vi "DAQmx Create Channel (AI-Strain-Rosette Strain Gage).vi"(0 "task in":refnum<k21>, 1 "maximum value":dbl=0.001 format="%0.7f", 2 "minimum value":dbl=-0.001 format="%0.7f", 5 "physical channels":tag, 7 "name to assign":string, 9 "rosette configuration":T1={"rosette type"=15968, "gage orientation"=0.0, "rosette measurements"=[15971]} {"rosette measurements" items=["Principal Strain 1"=15971, "Principal Strain 2"=15972, "Principal Strain Angle"=15973, "Cartesian Strain X"=15974, "Cartesian Strain Y"=15975, "Cartesian Shear Strain XY"=15976, "Maximum Shear Strain"=15977, "Maximum Shear Strain Angle"=15978]; "rosette type" items=["Rectangular Rosette"=15968, "Delta Rosette"=15969, "Tee Rosette"=15970]}, 11 "error in":errorcluster, 13 "bridge information":T2={"strain configuration"=10271, "lead wire resistance"=0.0, "voltage excitation source"=10200, "voltage excitation value"=2.5} {"voltage excitation source" items=["Internal"=10200, "External"=10167, "None"=10230]; "voltage excitation value" format="%0.2f"; "lead wire resistance" format="%0.2f"; "strain configuration" items=["Full Bridge I"=10183, "Full Bridge II"=10184, "Full Bridge III"=10185, "Half Bridge I"=10188, "Half Bridge II"=10189, "Quarter Bridge I"=10271, "Quarter Bridge II"=10272]}, 14 "strain gage information":T3={"gage factor"=2.0, "nominal gage resistance"=350.0, "poisson ratio"=0.3} {"poisson ratio" format="%0.2f"; "nominal gage resistance" format="%0.2f"; "gage factor" format="%0.2f"}) -> (4 "task out":refnum<k21>, 15 "error out":errorcluster)   [LabVIEW 2020]
doc: "Creates channels to measure two-dimensional strain using a rosette strain gage."
uses:
  nilvaiu.dll
panel:
  # "input limits"
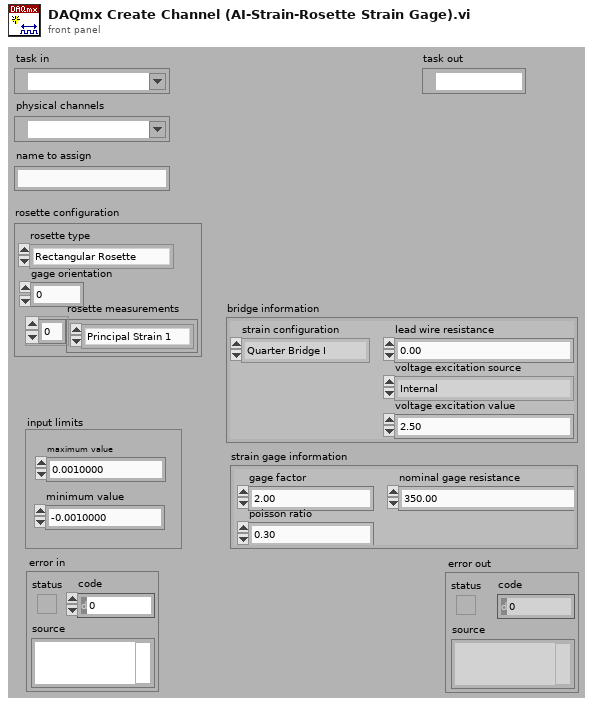
[diagram p1: front panel]
types:
  T1 = cluster{"rosette type":i32, "gage orientation":dbl, "rosette measurements":i32[]}
  T2 = cluster{"strain configuration":i32, "lead wire resistance":dbl, "voltage excitation source":i32, "voltage excitation value":dbl}
  T3 = cluster{"gage factor":dbl, "nominal gage resistance":dbl, "poisson ratio":dbl}
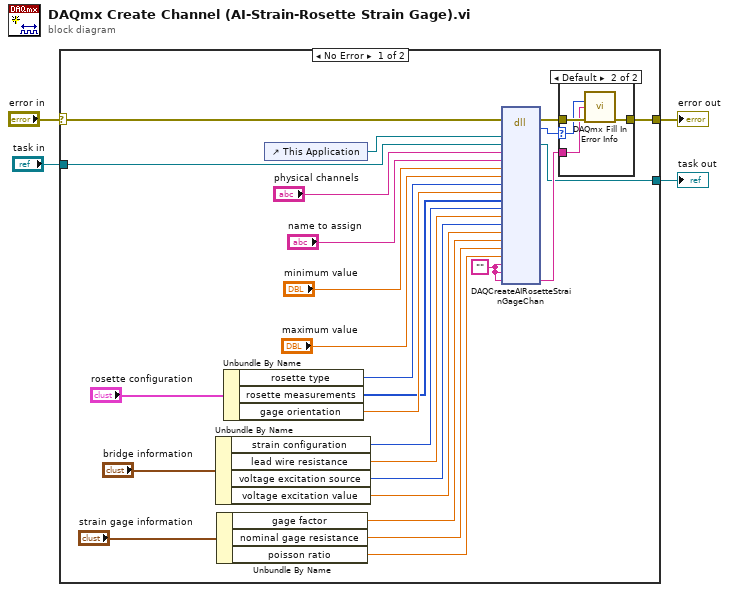
[diagram p0: block diagram]
diagram:
  n1 = case shown="No Error" "error in" {
    selector: "error in" -> [w20 w36]
    tunnel: [w19 w36] -> w4
    tunnel: "task in" -> [w22 w37]
    tunnel: [w18 w37] -> w1
    frame No Error {
      w5 = ""
      n2 = Unbundle By Name("bridge information") -> ("strain configuration"=w12:i32, "lead wire resistance"=w11:dbl, "voltage excitation source"=w10:i32, "voltage excitation value"=w9:dbl)
      n3 = Unbundle By Name("strain gage information") -> ("gage factor"=w8:dbl, "nominal gage resistance"=w7:dbl, "poisson ratio"=w6:dbl)
      n4 = Unbundle By Name("rosette configuration") -> ("rosette type"=w15:i32, "rosette measurements"=w13:i32[], "gage orientation"=w14:dbl)
      n5 = control-ref of="This Application"() -> (w21:refnum<vi>)
      n6 = dll-call lib="nilvaiu.*" fn="DAQCreateAIRosetteStrainGageChan"(error in=w20, "lvAppRef"=w21, "refObjPtr"=w22, "physicalChannelName"="physical channels", "channelNameIn"="name to assign", "minVal"="minimum value", "maxVal"="maximum value", "rosetteType"=w15, "gageOrientation"=w14, "rosetteMeasurementTypes"=w13, "strainConfig"=w12, "leadWireResist"=w11, "excitSource"=w10, "excitValue"=w9, "gageFactor"=w8, "nominalGageResist"=w7, "poissonRatio"=w6, "rawStrainChannelsOut"=w5, "calculatedRosetteChannelsOut"=w5, "extendedErrorInfo"=w5) -> (error out=w25:errorcluster, "return type"=w26:i32, "refObjPtr"=w18:refnum<k21>, "extendedErrorInfo"=w27:string)  [unwired: 19 in, 1 out]
      n7 = case shown="Default" w26 {
        selector: w26 -> [_ w33]
        tunnel: w25 -> [w31 w35]
        tunnel: [w31 w34] -> w19
        tunnel: w27 -> [_ w32]
        frame 0 {
        }
        frame Default {
          n8 = call "DAQmx Fill In Error Info.vi"("status code"=w33, "extended error info"=w32, "error in"=w35) -> ("error out"=w34:errorcluster)  [unwired: 1 in, 11 out]
        }
      }
    }
    frame Error {
    }
  }
  "error out" <- w4
  "task out" <- w1
